vi "To Binary.vi"(6 "byte order":T1(ring), 8 "error in (no error)":errorcluster, 11 "Double Float in":refnum<class "Abs_Complex Double Float.lvclass">) -> (0 "error out":errorcluster, 2 "Binary":string, 3 "Double Float out":refnum<class "Abs_Complex Double Float.lvclass">)   [LabVIEW 2021, in "Abs_Complex Double Float.lvclass"]
uses:
  Abs_Complex Double Float.lvclass
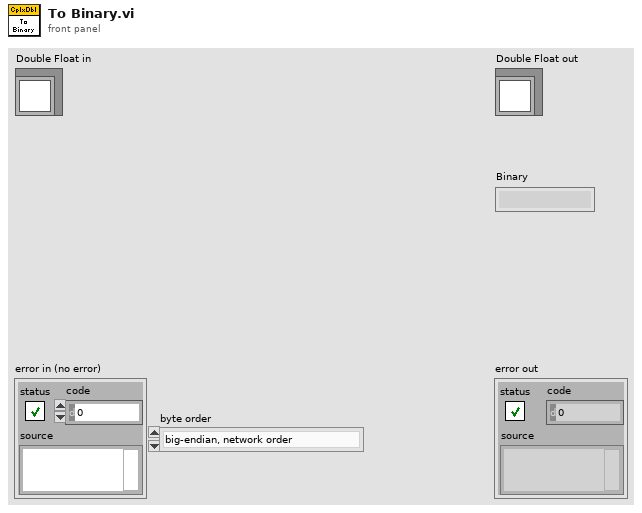
[diagram p1: front panel]
types:
  T1 = enum16{"big-endian, network order", "native, host order", "little-endian"}
  T2 = typedef "Abs_Complex Double Float.lvclass/Type.ctl" = cdb
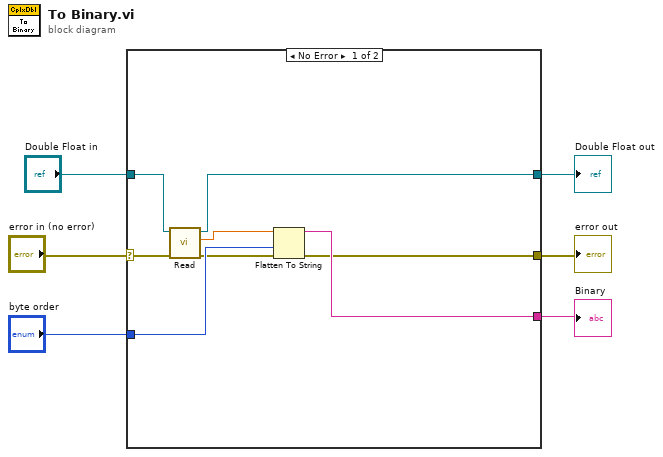
[diagram p0: block diagram]
diagram:
  n1 = case shown="No Error" "error in (no error)" {
    selector: "error in (no error)" -> [w11 w15]
    tunnel: [w12 w15] -> w3
    tunnel: [w8 w16] -> w2
    tunnel: "byte order" -> [w13 _]
    tunnel: "Double Float in" -> [w9 w16]
    tunnel: [w14 _] -> w1
    frame No Error {
      n2 = call-dynamic "Read.vi"("error in (no error)"=w11, "Double Float.lvclass_340760 in"=w9) -> ("error out"=w7:errorcluster, "Value"=w10:T2, "Double Float.lvclass_340760 out"=w8:refnum<class "Abs_Complex Double Float.lvclass">)  [unwired: 7 in]
      n3 = Flatten To String(anything=w10, byte order (0:big-endian, network order)=w13, error in (no error)=w7) -> (data string=w14:string, error out=w12:errorcluster)  [unwired: 1 in, 1 out]
    }
    frame Error {
    }
  }
  "error out" <- w3
  "Double Float out" <- w2
  "Binary" <- w1
